vi "run.vi"(8 "error in (no error)":errorcluster, 11 "DL090503StimulatorScaffold in":refnum<class "StimulatorAK101022TCP.lvclass">) -> (0 "error out":errorcluster, 3 "DL090503StimulatorScaffold out":refnum<class "StimulatorAK101022TCP.lvclass">)   [LabVIEW 2010, in "StimulatorAK101022TCP.lvclass"]
uses:
  StimulatorAK101022TCP.lvclass
  main/labview_source/controls/undock_button.ctl
  StimulatorDL090503Scaffold/StimulatorDL090503Scaffold/StimulatorDL090503Scaffold.lvclass
  StimulatorAK101022TCP.lvclass/StimulatorAK101022TCP.ctl
  StringGenerator/GenericStringGenerator/GenericStringGenerator/GenericStringGenerator.lvclass
  common/classes/ErrorController/ErrorController/class_data.vi
  common/classes/ErrorController/ErrorController/ErrorController.lvclass
  GenericStimulator/GenericStimulator/GenericStimulator.lvclass
panel:
  in  "button:undock":T1
  in  "settings":string(combo)="user-defined"
  in  "load settings":bool
  in  "save settings":bool
  in  "Tab Control":enum32{"User", "Debug", "About"}(tab)
  in  "modify":bool
  out "connected":bool
  in  "connect":bool
  in  "test":bool
  in  "TCP Signal":string
  in  "offset":dbl[unit]
  in  "duty cycle":dbl[unit]=1.0
  in  "repetitions":i32=1
  in  "rerandomize automatically":bool
  out "finished?":bool
  # "application"
  # "StimulatorDL090503\n\nImplemented by:\nAndreas Keller, ETH Zurich"
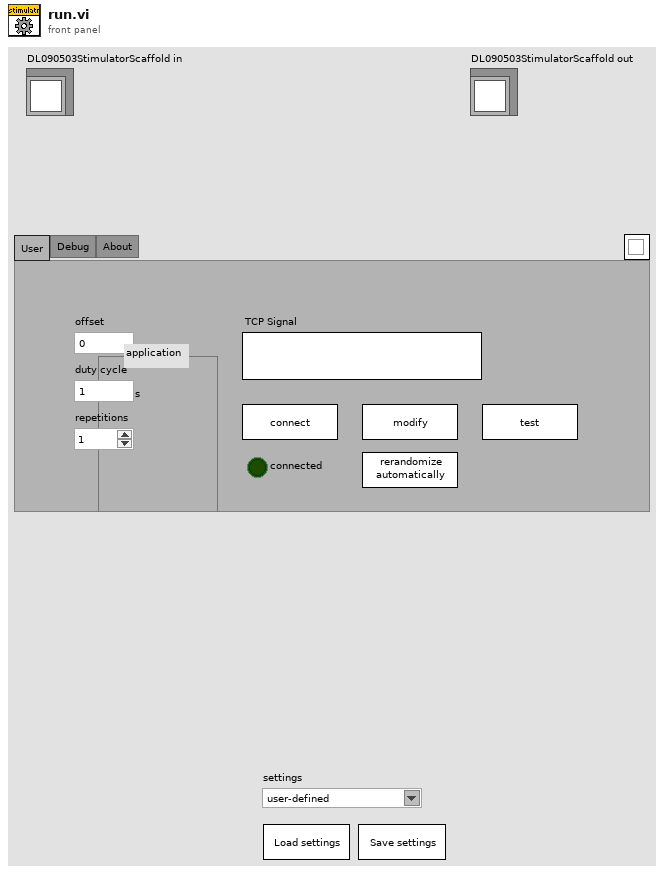
[diagram p1: front panel]
types:
  T1 = typedef "undock_button.ctl" = bool
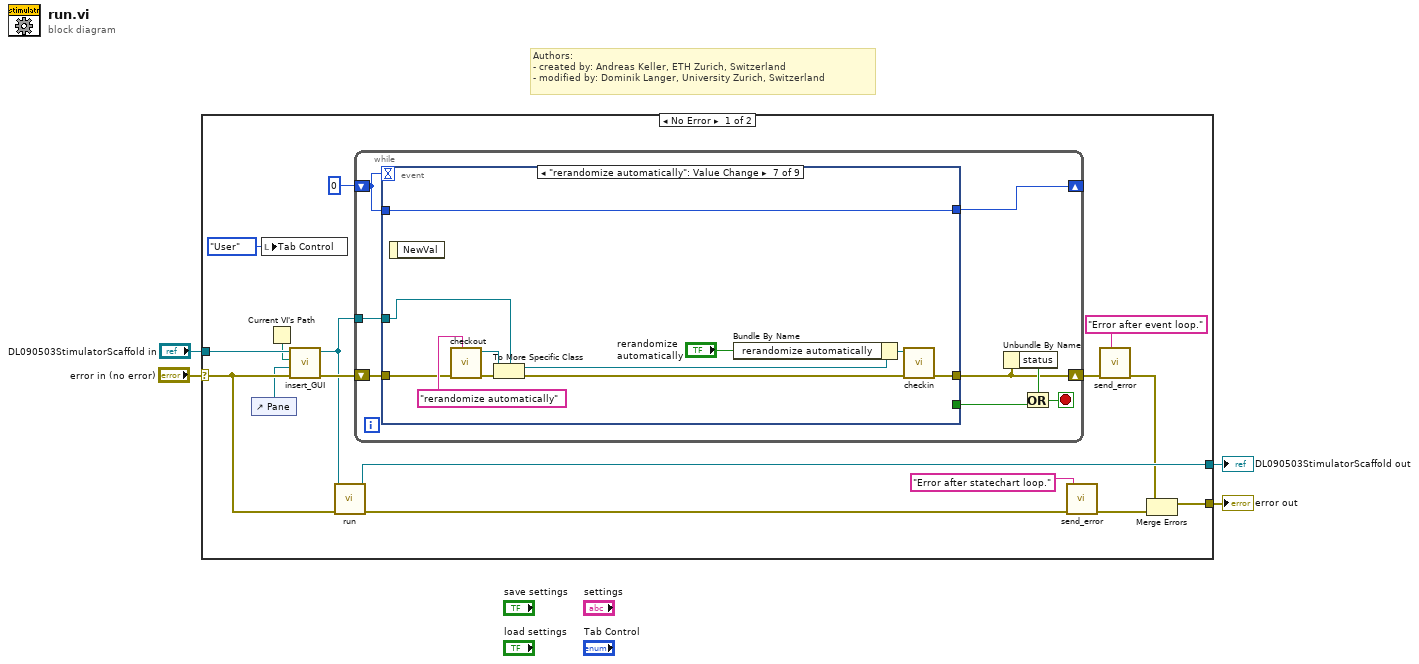
[diagram p0: block diagram]
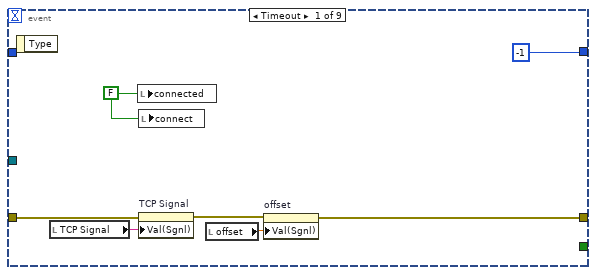
[diagram p2: hidden frame]
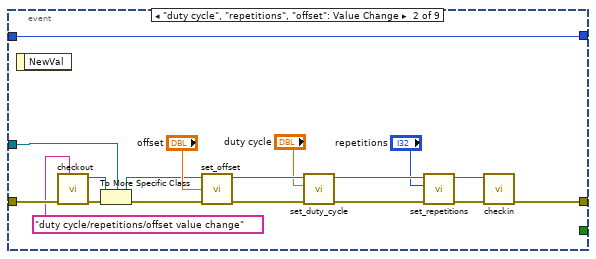
[diagram p3: hidden frame]
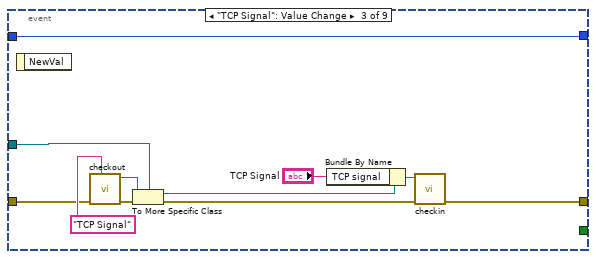
[diagram p4: hidden frame]
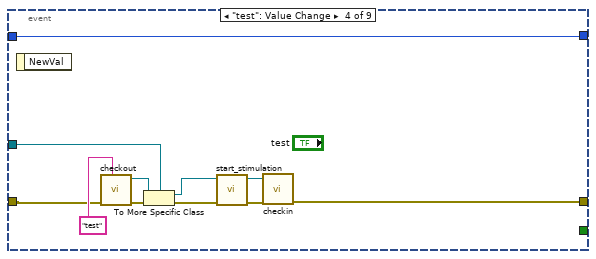
[diagram p5: hidden frame]
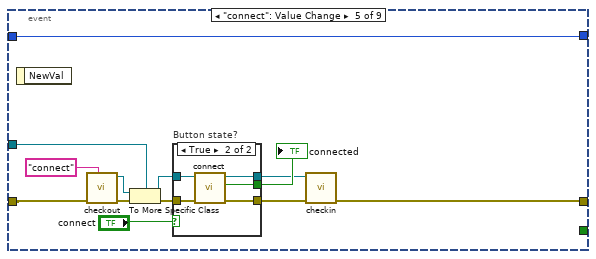
[diagram p6: hidden frame]
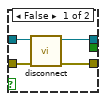
[diagram p7: hidden frame]
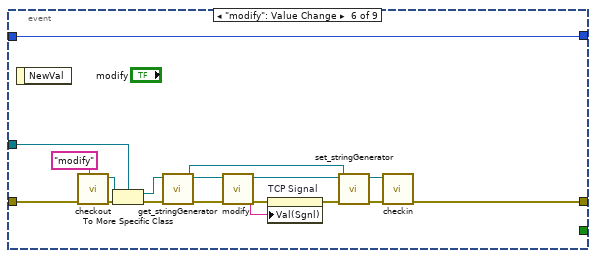
[diagram p8: hidden frame]
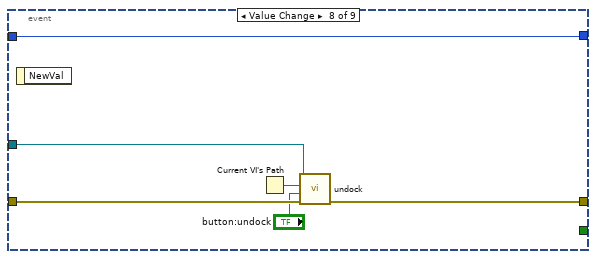
[diagram p9: hidden frame]
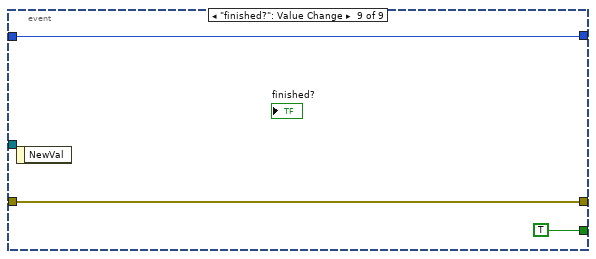
[diagram p10: hidden frame]
diagram:
  # "Authors: \n- created by: Andreas Keller, ETH Zurich, Switzerland\n- modified by: Dominik Langer, University Zurich, Switzerland"
  n1 = case shown="No Error" "error in (no error)" {
    selector: "error in (no error)" -> [w10 w137]
    tunnel: "DL090503StimulatorScaffold in" -> [w11 w136]
    tunnel: [w19 w137] -> w4
    tunnel: [w18 w136] -> w3
    frame No Error {
      n2 = control-ref of="Pane"() -> (w8:refnum<vi>)
      n3 = local write "Tab Control"(enum32{"User", "Debug", "About"}."User" ("Tab Control")) -> ()
      n4 = Current VI's Path() -> (path=w9:path)
      n5 = call-dynamic "insert_GUI.vi"("error in (no error)"=w10, "Pane"=w8, "VI path"=w9, "GenericComponent in"=w11) -> ("error out"=w7:errorcluster, "GenericComponent out"=w6:refnum<class "StimulatorAK101022TCP.lvclass">)  [unwired: 6 in]
      n6 = call-parent "run.vi"("error in (no error)"=w10, "DL090503StimulatorScaffold in"=w6) -> ("error out"=w14:errorcluster, "DL090503StimulatorScaffold out"=w18:refnum<class "StimulatorAK101022TCP.lvclass">)  [unwired: 8 in]
      n7 = while {
        shift-right: [w27] -> _
        shift-left: 0 -> [w23]
        shift-right: [w21] -> w17
        shift-left: w7 -> [w28]
        tunnel: w6 -> [w22]
        stop <- w26 stop-if-true
        n8 = event shown="[6] \"rerandomize automatically\": Value Change" {
          selector: _ -> [_ _ _ _ _ _ _ _ _]
          dyn-events: _ -> [_ _ _ _ _ _ _ _ _]
          timeout: w23 -> [_ _ _ _ _ _ _ _ _]
          tunnel: [w30 w37 w58 w66 w84 w100 w117 w129 w135] -> w21
          tunnel: w28 -> [w33 w44 w61 w72 w86 w110 w118 w130 w135]
          tunnel: w23 -> [_ w46 w54 w65 w78 w115 w126 w132 w133]
          tunnel: [-1 w46 w54 w65 w78 w115 w126 w132 w133] -> w27
          tunnel: [_ _ _ _ _ _ _ _ TRUE] -> w24
          tunnel: w22 -> [_ w36 w60 w70 w85 w109 w119 w131 _]
          event Timeout {
            w34 = FALSE
            n9 = event-data() -> ()  [unwired: 1 in, 1 out]
            n10 = local read "TCP Signal"() -> (w32:string)
            n11 = local write "connected"(w34) -> ()
            n12 = local write "connect"(w34) -> ()
            n13 = property on="TCP Signal" class="Str"(error in=w33, "Val(Sgnl)"=w32) -> (error out=w29:errorcluster)  [unwired: 1 in, 1 out]
            n14 = local read "offset"() -> (w31:dbl[unit])
            n15 = property on="offset" class="DigNum (strict)"(error in=w29, "Val(Sgnl)"=w31) -> (error out=w30:errorcluster)  [unwired: 1 in, 1 out]
          }
          event "duty cycle", "repetitions", "offset": Value Change {
            n16 = event-data() -> ()  [unwired: 1 in, 1 out]
            n17 = call "checkout.vi"("locked by?"="duty cycle/repetitions/offset value change", "error in (no error)"=w44) -> ("error out"=w43:errorcluster, "GenericStimulator out"=w42:refnum<class "GenericStimulator.lvclass">)  [unwired: 8 in]
            n18 = To More Specific Class(target class=w36, reference=w42, error in=w43) -> (specific class reference=w45:refnum<class "StimulatorAK101022TCP.lvclass">, error out=w40:errorcluster)
            n19 = call-dynamic "set_offset.vi"("error in (no error)"=w40, "offset"="offset", "DL090503StimulatorScaffold.lvclass in"=w45) -> ("error out"=w53:errorcluster, "DL090503StimulatorScaffold.lvclass out"=w51:refnum<class "StimulatorAK101022TCP.lvclass">)  [unwired: 7 in]
            n20 = call-dynamic "set_duty_cycle.vi"("error in (no error)"=w53, "duty cycle"="duty cycle", "DL090503StimulatorScaffold.lvclass in"=w51) -> ("error out"=w52:errorcluster, "DL090503StimulatorScaffold.lvclass out"=w50:refnum<class "StimulatorAK101022TCP.lvclass">)  [unwired: 7 in]
            n21 = call-dynamic "set_repetitions.vi"("error in (no error)"=w52, "repetitions"="repetitions", "DL090503StimulatorScaffold.lvclass in"=w50) -> ("error out"=w38:errorcluster, "DL090503StimulatorScaffold.lvclass out"=w39:refnum<class "StimulatorAK101022TCP.lvclass">)  [unwired: 7 in]
            n22 = call-dynamic "checkin.vi"("error in (no error)"=w38, "GenericStimulator in"=w39) -> ("error out"=w37:errorcluster)  [unwired: 8 in, 1 out]
          }
          event "TCP Signal": Value Change {
            n23 = event-data() -> ()  [unwired: 1 in, 1 out]
            n24 = call "checkout.vi"("locked by?"="TCP Signal", "error in (no error)"=w61) -> ("error out"=w64:errorcluster, "GenericStimulator out"=w63:refnum<class "GenericStimulator.lvclass">)  [unwired: 8 in]
            n25 = To More Specific Class(target class=w60, reference=w63, error in=w64) -> (specific class reference=w57:refnum<class "StimulatorAK101022TCP.lvclass">, error out=w59:errorcluster)
            n26 = Bundle By Name(cluster=w57, "TCP signal"="TCP Signal") -> (w56:refnum<class "StimulatorAK101022TCP.lvclass">)
            n27 = call-dynamic "checkin.vi"("error in (no error)"=w59, "GenericStimulator in"=w56) -> ("error out"=w58:errorcluster)  [unwired: 8 in, 1 out]
          }
          event "test": Value Change {
            n28 = event-data() -> ()  [unwired: 1 in, 1 out]
            n29 = call "checkout.vi"("locked by?"="test", "error in (no error)"=w72) -> ("error out"=w75:errorcluster, "GenericStimulator out"=w74:refnum<class "GenericStimulator.lvclass">)  [unwired: 8 in]
            n30 = To More Specific Class(target class=w70, reference=w74, error in=w75) -> (specific class reference=w69:refnum<class "StimulatorAK101022TCP.lvclass">, error out=w71:errorcluster)
            n31 = call-dynamic "start_stimulation.vi"("error in (no error)"=w71, "DL090503StimulatorScaffold in"=w69) -> ("error out"=w68:errorcluster, "DL090503StimulatorScaffold out"=w67:refnum<class "StimulatorAK101022TCP.lvclass">)  [unwired: 8 in]
            n32 = call-dynamic "checkin.vi"("error in (no error)"=w68, "GenericStimulator in"=w67) -> ("error out"=w66:errorcluster)  [unwired: 8 in, 1 out]
          }
          event "connect": Value Change {
            n33 = event-data() -> ()  [unwired: 1 in, 1 out]
            n34 = call "checkout.vi"("locked by?"="connect", "error in (no error)"=w86) -> ("error out"=w88:errorcluster, "GenericStimulator out"=w76:refnum<class "GenericStimulator.lvclass">)  [unwired: 8 in]
            n35 = To More Specific Class(target class=w85, reference=w76, error in=w88) -> (specific class reference=w81:refnum<class "StimulatorAK101022TCP.lvclass">, error out=w83:errorcluster)
            n36 = case "Button state?" shown="True" "connect" {
              tunnel: w83 -> [w92 w97]
              tunnel: [w91 w96] -> w82
              tunnel: w81 -> [w89 w95]
              tunnel: [_ w94] -> w80
              tunnel: [w90 w93] -> w79
              frame False {
                n37 = call-dynamic "disconnect.vi"("error in (no error)"=w92, "StimulatorAK101022TCP in"=w89) -> ("error out"=w91:errorcluster, "StimulatorAK101022TCP out"=w90:refnum<class "StimulatorAK101022TCP.lvclass">)  [unwired: 8 in]
              }
              frame True {
                n38 = call-dynamic "connect.vi"("error in (no error)"=w97, "StimulatorAK101022TCP in"=w95) -> ("error out"=w96:errorcluster, "connected"=w94:bool, "StimulatorAK101022TCP out"=w93:refnum<class "StimulatorAK101022TCP.lvclass">)  [unwired: 7 in]
              }
            }
            "connected" <- w80
            n39 = call-dynamic "checkin.vi"("error in (no error)"=w82, "GenericStimulator in"=w79) -> ("error out"=w84:errorcluster)  [unwired: 8 in, 1 out]
          }
          event "modify": Value Change {
            n40 = event-data() -> ()  [unwired: 1 in, 1 out]
            n41 = call "checkout.vi"("locked by?"="modify", "error in (no error)"=w110) -> ("error out"=w113:errorcluster, "GenericStimulator out"=w111:refnum<class "GenericStimulator.lvclass">)  [unwired: 8 in]
            n42 = To More Specific Class(target class=w109, reference=w111, error in=w113) -> (specific class reference=w108:refnum<class "StimulatorAK101022TCP.lvclass">, error out=w107:errorcluster)
            n43 = call-dynamic "get_stringGenerator.vi"("error in (no error)"=w107, "StimulatorAK101022TCP in"=w108) -> ("error out"=w106:errorcluster, "stringGenerator"=w105:refnum<class "GenericStringGenerator.lvclass">, "StimulatorAK101022TCP out"=w98:refnum<class "StimulatorAK101022TCP.lvclass">)  [unwired: 7 in]
            n44 = call-dynamic "modify.vi"("error in (no error)"=w106, "GenericStringGenerator in"=w105) -> ("error out"=w102:errorcluster, "String"=w114:string, "GenericStringGenerator out"=w104:refnum<class "GenericStringGenerator.lvclass">)  [unwired: 7 in]
            n45 = property on="TCP Signal" class="Str"(error in=w102, "Val(Sgnl)"=w114) -> (error out=w101:errorcluster)  [unwired: 1 in, 1 out]
            n46 = call-dynamic "set_stringGenerator.vi"("error in (no error)"=w101, "subcomponents.stringGenerator"=w104, "StimulatorAK101022TCP in"=w98) -> ("error out"=w103:errorcluster, "StimulatorAK101022TCP out"=w99:refnum<class "StimulatorAK101022TCP.lvclass">)  [unwired: 7 in]
            n47 = call-dynamic "checkin.vi"("error in (no error)"=w103, "GenericStimulator in"=w99) -> ("error out"=w100:errorcluster)  [unwired: 8 in, 1 out]
          }
          event "rerandomize automatically": Value Change {
            n48 = event-data() -> ()  [unwired: 1 in, 1 out]
            n49 = call "checkout.vi"("locked by?"="rerandomize automatically", "error in (no error)"=w118) -> ("error out"=w125:errorcluster, "GenericStimulator out"=w124:refnum<class "GenericStimulator.lvclass">)  [unwired: 8 in]
            n50 = To More Specific Class(target class=w119, reference=w124, error in=w125) -> (specific class reference=w121:refnum<class "StimulatorAK101022TCP.lvclass">, error out=w122:errorcluster)
            n51 = Bundle By Name(cluster=w121, "rerandomize automatically"="rerandomize automatically") -> (w120:refnum<class "StimulatorAK101022TCP.lvclass">)
            n52 = call-dynamic "checkin.vi"("error in (no error)"=w122, "GenericStimulator in"=w120) -> ("error out"=w117:errorcluster)  [unwired: 8 in, 1 out]
          }
          event Value Change {
            n53 = event-data() -> ()  [unwired: 1 in, 1 out]
            n54 = Current VI's Path() -> (path=w127:path)
            n55 = call-dynamic "undock.vi"("error in (no error)"=w130, "undock?"="button:undock", "VI path"=w127, "GenericComponent in"=w131) -> ("error out"=w129:errorcluster)  [unwired: 6 in, 1 out]
          }
          event "finished?": Value Change {
            n56 = event-data() -> ()  [unwired: 1 in, 1 out]
          }
        }
        n57 = Unbundle By Name(w21) -> ("status"=w25:bool)
        n58 = Or(x=w25, y=w24) -> (x .or. y?=w26:bool)
      }
      n59 = call "send_error.vi"("additional message"="Error after statechart loop.", "error in (no error)"=w14) -> ("error out"=w13:errorcluster)  [unwired: 9 in]
      n60 = call "send_error.vi"("additional message"="Error after event loop.", "error in (no error)"=w17) -> ("error out"=w16:errorcluster)  [unwired: 9 in]
      n61 = Merge Errors(w16, w13) -> (w19:errorcluster)
    }
    frame Error {
    }
  }
  "error out" <- w4
  "DL090503StimulatorScaffold out" <- w3
